vi "setAO_DC.vi"(8 "error in (no error)":errorcluster, 9 "DC (V)":dbl, 10 "AO Channel":i32=1 min=1 max=16, 11 "Instrument.LockinAPI in":refnum<class "Instrument.LockinAPI.lvclass">) -> (0 "error out":errorcluster, 3 "Instrument.LockinAPI out":refnum<class "Instrument.LockinAPI.lvclass">)   [LabVIEW 2019, in "Instrument.LockinAPI.lvclass"]
doc: "API to configure an AO DC offset.\n\nSpecify which channel you want to change and the value you want to set.\n\nIf address=\"\", this API reads from localhost\nIf address is remote lockin, you need to add this computer to allowed whitelist on the lockin computer you are trying to access."
uses:
  Instrument.LockinAPI.lvclass
  Typedefs/LockinAPI.Commands--Enum.ctl
  Typedefs/LockinAPI.AO_DC--cluster.ctl
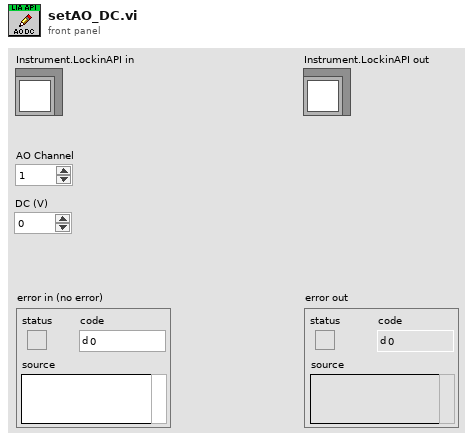
[diagram p1: front panel]
types:
  T1 = typedef "Instrument.LockinAPI.lvclass/LockinAPI.AO_DC--cluster.ctl" = cluster{"Channel":i32, "DC":dbl}
  T2 = typedef "Instrument.LockinAPI.lvclass/LockinAPI.Commands--Enum.ctl" = enum16{"setAI", "setAO", "setAO_Amplitude", "setAO_DC", "setAO_Frequency", "setAO_Phase", "setAO_Function", "setREF", "setREF_Frequency", "setREF_Phase", "setREF_TC", "setREF_Roll-Off", "setDAQ", "setSampling", "setOffset", "setState", "getState", "getAO", "getAI", "getResults", "getSampling", "getAOconfig", "getREFconfig", "setInputGain", "setOutputGain", "getInputGain", "getOutputGain", "setSweep", "setSweep_Time", "setSweep_Table", "getStatus", "getSweepResults", "getSweepWaveforms", "startSweep", "stopSweep"}
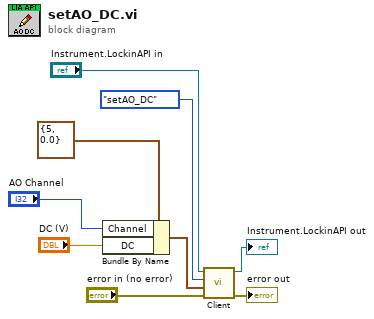
[diagram p0: block diagram]
diagram:
  n1 = Bundle By Name(cluster=T1 {"Channel"=5, "DC"=0.0} ("setAO_DC"), "Channel"="AO Channel", "DC"="DC (V)") -> (w9:T1)
  n2 = call-dynamic "Client.vi"("error in (no error)"="error in (no error)", "Data in"=w9, "Command in"=LockinAPI.Commands--Enum."setAO_DC" ("Command"), "Instrument in"="Instrument.LockinAPI in") -> ("error out"=→"error out":errorcluster, "Instrument out"=→"Instrument.LockinAPI out":refnum<class "Instrument.LockinAPI.lvclass">)  [unwired: 4 in, 2 out]
